vi "LaserBatchMode.vi"(10 "Batch Size":dbl, 11 "client handle in":T1) -> (3 "client handle out":T1)   [LabVIEW 2020]
uses:
  <vilib>/httpClient/ClientHandle.ctl
  <vilib>/httpClient/LabVIEWHTTPClient.lvlib
  <vilib>/wsapi/NI_WebServices.lvlib
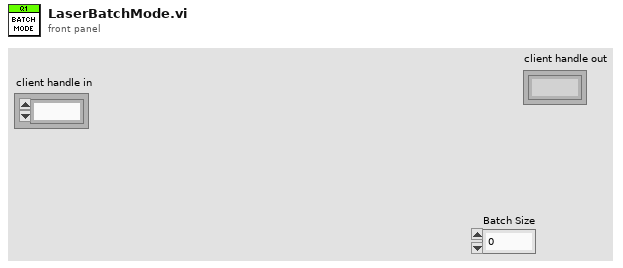
[diagram p1: front panel]
types:
  T1 = typedef "LabVIEWHTTPClient.lvlib/ClientHandle.ctl" = refnum<k1>
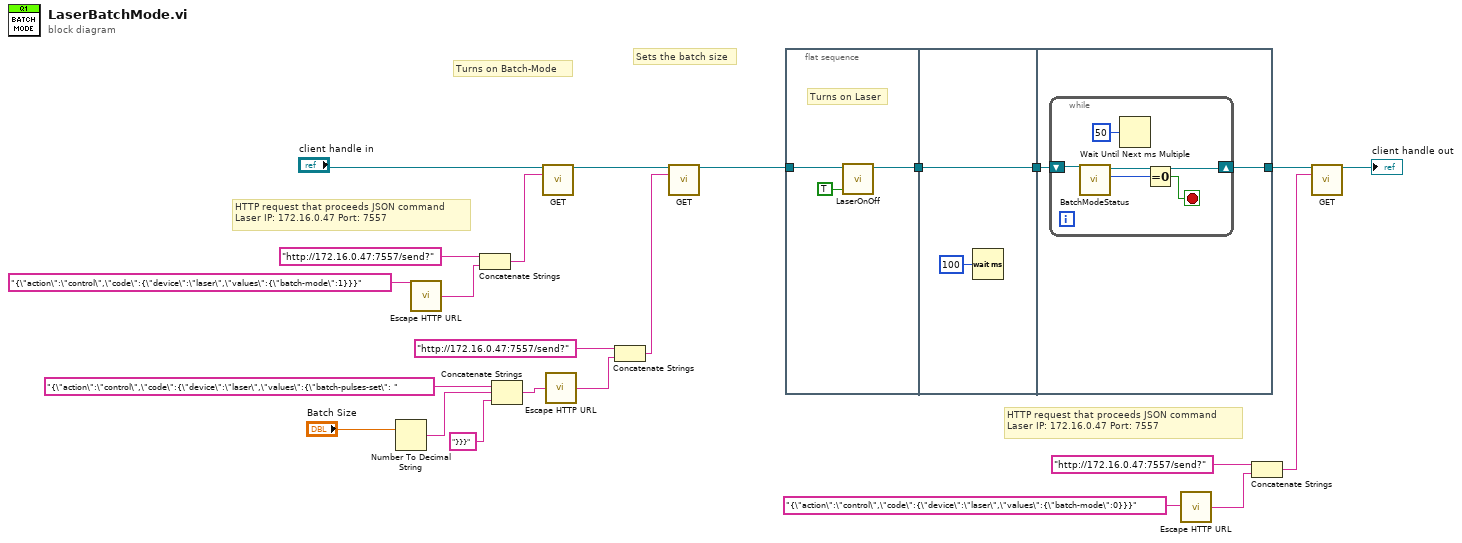
[diagram p0: block diagram]
diagram:
  # "HTTP request that proceeds JSON command\nLaser IP: 172.16.0.47 Port: 7557"
  # "Sets the batch size"
  # "Turns on Batch-Mode"
  # "HTTP request that proceeds JSON command\nLaser IP: 172.16.0.47 Port: 7557"
  n1 = Number To Decimal String(number="Batch Size") -> (decimal integer string=w13:string)  [unwired: 1 in]
  n2 = call <vilib>:"Escape HTTP URL.vi"("unescaped string in"="{\"action\":\"control\",\"code\":{\"device\":\"laser\",\"values\":{\"batch-mode\":1}}}" ("JSON command")) -> ("escaped string out"=w21:string)
  n3 = Concatenate Strings("http://172.16.0.47:7557/send?", w21) -> (w23:string)
  n4 = Concatenate Strings("{\"action\":\"control\",\"code\":{\"device\":\"laser\",\"values\":{\"batch-pulses-set\": " ("JSON command"), w13, "}}}" ("string")) -> (w17:string)
  n5 = call <vilib>:"GET.vi"("client handle"="client handle in", "url"=w23) -> ("client handle out"=w20:T1)  [unwired: 10 in, 3 out]
  n6 = call <vilib>:"Escape HTTP URL.vi"("unescaped string in"=w17) -> ("escaped string out"=w18:string)
  n7 = Concatenate Strings("http://172.16.0.47:7557/send?", w18) -> (w15:string)
  n8 = call <vilib>:"GET.vi"("client handle"=w20, "url"=w15) -> ("client handle out"=w4:T1)  [unwired: 10 in, 3 out]
  n9 = flat-sequence {
    tunnel: w4 -> [w25]
    tunnel: [w24] -> w2
    tunnel: [w27] -> w3
    tunnel: w2 -> [w27]
    tunnel: [w30] -> w1
    tunnel: w3 -> [w29]
    frame #0 {
      # "Turns on Laser"
      n10 = call "LaserOnOff.vi"("Laser on/off"=TRUE, "client handle in"=w25) -> ("client handle out"=w24:T1)  [unwired: 8 in, 1 out]
    }
    frame #1 {
      n11 = Wait (ms)(milliseconds to wait=u32 100) -> ()  [unwired: 1 out]
    }
    frame #2 {
      n12 = while {
        shift-right: [w34] -> w30
        shift-left: w29 -> [w35]
        stop <- w33 stop-if-true
        n13 = call "BatchModeStatus.vi"("client handle in"=w35) -> ("batch-mode-pulses-remaining"=w32:i32, "client handle out"=w34:T1)  [unwired: 8 in, 1 out]
        n14 = Wait Until Next ms Multiple(millisecond multiple=u32 50) -> ()  [unwired: 1 out]
        n15 = Equal To 0?(x=w32) -> (x = 0?=w33:bool)
      }
    }
  }
  n16 = call <vilib>:"Escape HTTP URL.vi"("unescaped string in"="{\"action\":\"control\",\"code\":{\"device\":\"laser\",\"values\":{\"batch-mode\":0}}}" ("JSON command")) -> ("escaped string out"=w9:string)
  n17 = Concatenate Strings("http://172.16.0.47:7557/send?", w9) -> (w8:string)
  n18 = call <vilib>:"GET.vi"("client handle"=w1, "url"=w8) -> ("client handle out"=→"client handle out":T1)  [unwired: 10 in, 3 out]
